vi "Init T-Cube.vi"(8 "entrée d'erreur (pas d'erreur)":errorcluster, 10 "SerialNumber":string, 11 "Refnum de .NET en entrée":refnum<k24>) -> (0 "sortie d'erreur":errorcluster, 3 "Refnum de .NET en sortie":refnum<k24>)   [LabVIEW 2026]
uses:
  C:/Users/flepetit/Desktop/Projet BTS Photonique/Thorlabs.MotionControl.Controls.dll
  Thorlabs.MotionControl.Controls.dll
  C:/Users/flepetit/Desktop/Projet BTS Photonique/Thorlabs.MotionControl.TCube.PiezoCLI.dll
  Thorlabs.MotionControl.TCube.PiezoCLI.dll
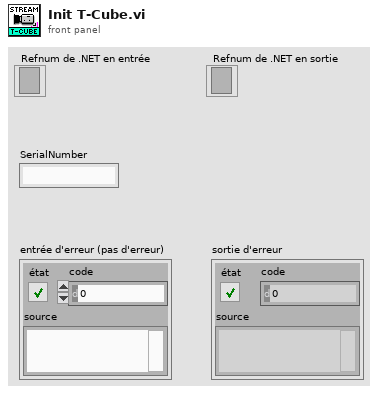
[diagram p1: front panel]
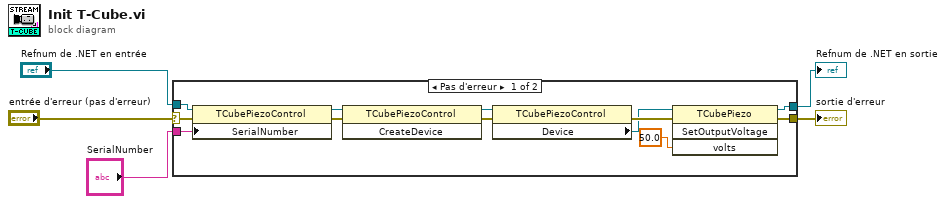
[diagram p0: block diagram]
diagram:
  n1 = case shown="Pas d'erreur" "entrée d'erreur (pas d'erreur)" {
    selector: "entrée d'erreur (pas d'erreur)" -> [w6 w18]
    tunnel: "SerialNumber" -> [w17 _]
    tunnel: "Refnum de .NET en entrée" -> [w16 _]
    tunnel: [w9 w18] -> w3
    tunnel: [w8 _] -> w2
    frame No Error {
      n2 = property class="TCubePiezoControl"(reference=w16, error in=w6, "SerialNumber"=w17) -> (reference out=w12:refnum<k24>, error out=w13:errorcluster)
      n3 = invoke class="TCubePiezoControl" method="CreateDevice"(reference=w12, error in=w13) -> (reference out=w14:refnum<k24>, error out=w15:errorcluster)  [unwired: 1 in, 1 out]
      n4 = property class="TCubePiezoControl"(reference=w14, error in=w15) -> (error out=w11:errorcluster, "Device"=w10:refnum<k24>)  [unwired: 1 out]
      n5 = invoke class="TCubePiezo" method="SetOutputVoltage"(reference=w10, error in=w11, "volts"=50.0) -> (reference out=w8:refnum<k24>, error out=w9:errorcluster)  [unwired: 1 in, 2 out]
    }
    frame Error {
    }
  }
  "Refnum de .NET en sortie" <- w2
  "sortie d'erreur" <- w3
